vi "ShutdownReceived.vi"(8 "error in (no error)":errorcluster, 11 "Shutdown?":bool) -> (0 "error out":errorcluster)   [LabVIEW 2017, in "communicateMLC.lvlib"]
uses:
  communicateMLC.lvlib
  programControl/Queue/TypeDefs/message.ctl
  programControl/programControl.lvlib
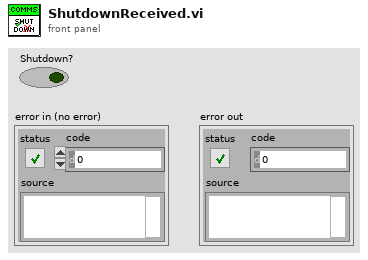
[diagram p1: front panel]
types:
  T1 = typedef "programControl.lvlib/message.ctl" = cluster{"calling module":string, "message":string, "Data":variant}
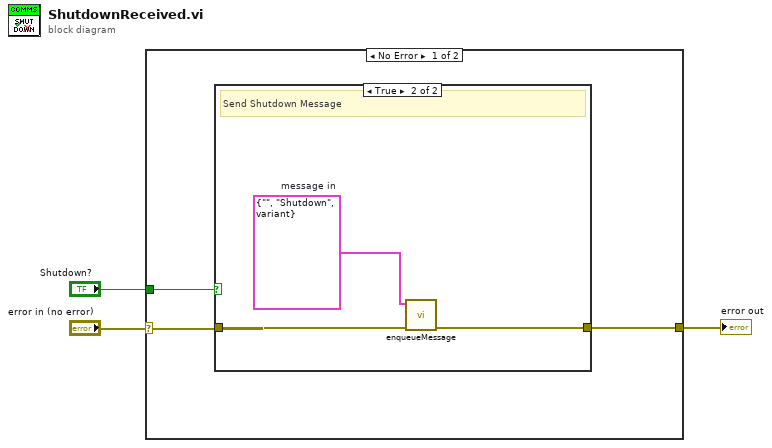
[diagram p0: block diagram]
diagram:
  n1 = case shown="No Error" "error in (no error)" {
    selector: "error in (no error)" -> [w4 w11]
    tunnel: "Shutdown?" -> [w6 _]
    tunnel: [w5 w11] -> w2
    frame No Error {
      n2 = case shown="True" w6 {
        tunnel: w4 -> [w7 w10]
        tunnel: [w7 w9] -> w5
        frame False {
          # "Do Nothing"
        }
        frame True {
          w8 = T1 {"calling module"="", "message"="Shutdown", "Data"=variant}  # message in
          # "Send Shutdown Message"
          n3 = call "enqueueMessage.vi"("error in (no error)"=w10, "element"=w8) -> ("error out"=w9:errorcluster)  [unwired: 9 in]
        }
      }
    }
    frame Error {
    }
  }
  "error out" <- w2
